vi "deferPanel.vi"(7 "EnumDeferPanel":T1, 8 "errorIn":errorcluster) -> (0 "error out":errorcluster)   [LabVIEW 2011]
uses:
  enumDeferPanelUpdate.ctl
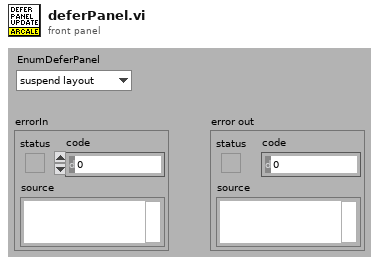
[diagram p1: front panel]
types:
  T1 = typedef "enumDeferPanelUpdate.ctl" = enum16{"suspend layout", "resume layout"}
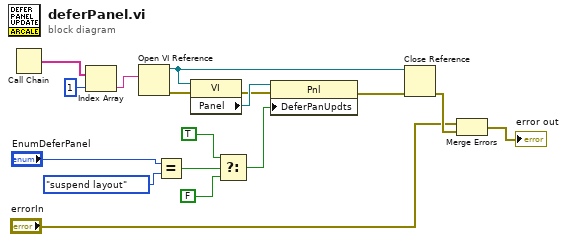
[diagram p0: block diagram]
diagram:
  n1 = Call Chain() -> (call chain=w17:string[])
  n2 = Index Array(array=w17, index=1) -> (element=w15:string)
  n3 = Open VI Reference(vi path=w15) -> (vi reference=w12:refnum<vi>, error out=w10:errorcluster)  [unwired: 1 in, 4 out]
  n4 = Equal?(x="EnumDeferPanel", y=enumDeferPanelUpdate."suspend layout") -> (x = y?=w6:bool)
  n5 = property class="VI"(reference=w12, error in=w10) -> (error out=w13:errorcluster, "Panel"=w14:refnum<vi>)  [unwired: 1 out]
  n6 = Select(t=TRUE, s=w6, f=FALSE) -> (s? t:f=w5:bool)
  n7 = property class="Pnl"(reference=w14, error in=w13, "DeferPanUpdts"=w5) -> (error out=w11:errorcluster)  [unwired: 1 out]
  n8 = Close Reference(reference=w12, error in (no error)=w11) -> (error out=w2:errorcluster)
  n9 = Merge Errors("errorIn", w2) -> (→"error out":errorcluster)
